vi "MG3700 Indentification Query.vi"(0 "VISA In":refnum<visa-resource-name>, 1 "Error in (no error)":errorcluster) -> (2 "VISA Out":refnum<visa-resource-name>, 3 "Identify Response":string, 4 "Error code":i32, 5 "Error out":errorcluster)   [LabVIEW 2015]
doc: "sFunction: Returns product identification information, including the manufacturer' name and model name."
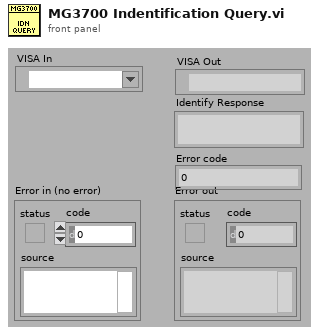
[diagram p1: front panel]
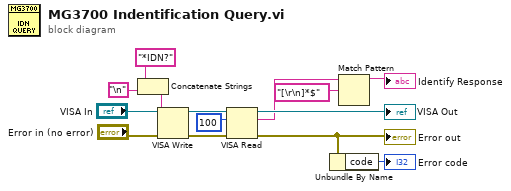
[diagram p0: block diagram]
diagram:
  n1 = Concatenate Strings("*IDN?" ("_Command"), "\n") -> (w5:string)
  n2 = VISA Write(VISA resource name="VISA In", write buffer=w5, error in (no error)="Error in (no error)") -> (VISA resource name out=w12:refnum<visa-resource-name>, error out=w11:errorcluster)  [unwired: 1 out]
  n3 = VISA Read(VISA resource name=w12, byte count=u32 100 ("byte count (0)"), error in (no error)=w11) -> (VISA resource name out=→"VISA Out":refnum<visa-resource-name>, read buffer=w2:string, error out=w8:errorcluster)  [unwired: 1 out]
  "Error out" <- w8
  n4 = Unbundle By Name(w8) -> ("code"=→"Error code":i32)
  n5 = Match Pattern(string=w2, regular expression="[\r\n]*$" ("search string")) -> (before substring=→"Identify Response":string)  [unwired: 1 in, 3 out]
